vi "AssertValueByArrayTags.vi"(0 "VI Reference In":refnum<vi>, 1 "Test Label":string, 2 "delimiter (>>)":string=">>", 3 "Assert Only? (F)":bool, 5 "Control Path":string, 7 "Focus Item Tag":string[](array[string]), 11 "Error In":errorcluster, 12 "Assert Interval(10 ms)":u32=10, 13 "Timeout(5 sec)":dbl=5.0) -> (4 "VI Reference Out":refnum<vi>, 6 "Asserted Value":string[](array[string]), 15 "Error Out":errorcluster)   [LabVIEW 2016, in "Drona.lvlib" / "AssertControlValue.lvlib" / "AssertTree.lvlib"]
doc: "Asserts if the array of focus item tags for the multi-select tree control are equal.\n\nThe input control name is given as a string , incase of path, use delimiters inbetween the path.\nThis VI gets the value of the control, untill the value is equal to the input value."
uses:
  AssertTree.lvlib
  Get/GetControlRef/GetControlRefByPath.vi
  <vilib>/addons/_JKI Toolkits/Caraya/classes/Assert/Assert Equal Value_Variant.vi
  Get/GetControlRef/GetControlRef.lvlib
  <vilib>/addons/_JKI Toolkits/Caraya/classes/Assert/Assert.lvclass
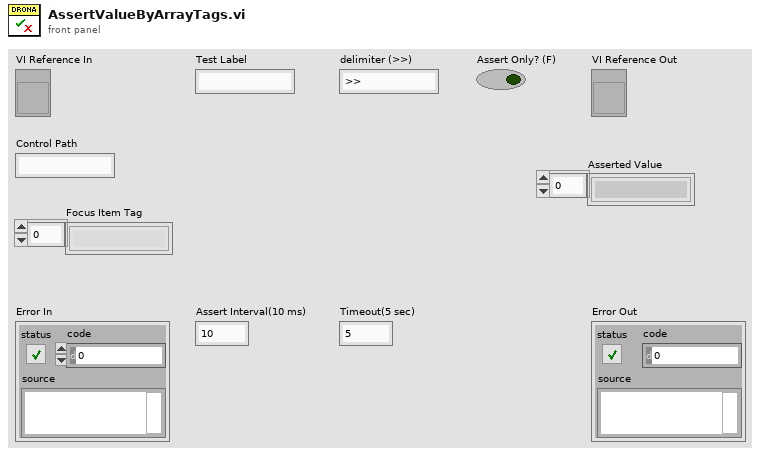
[diagram p1: front panel]
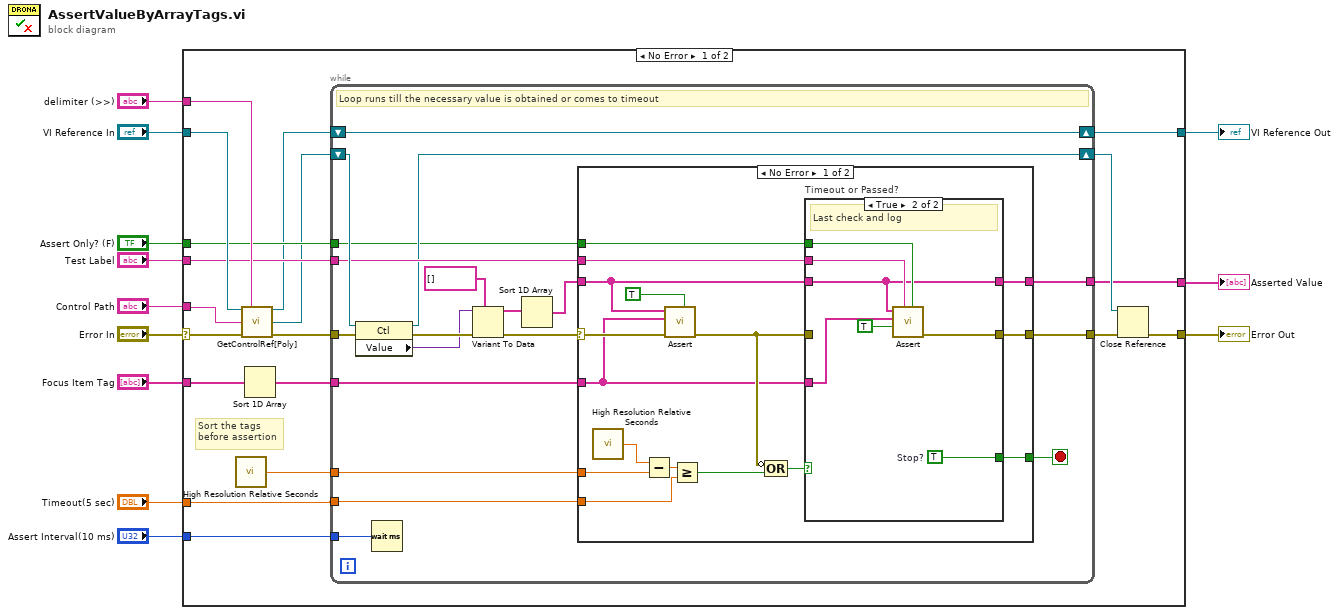
[diagram p0: block diagram]
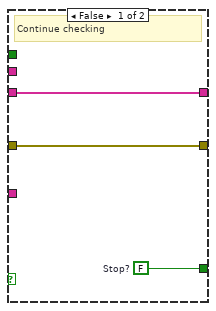
[diagram p2: hidden frame]
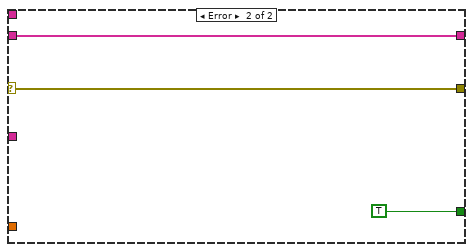
[diagram p3: hidden frame]
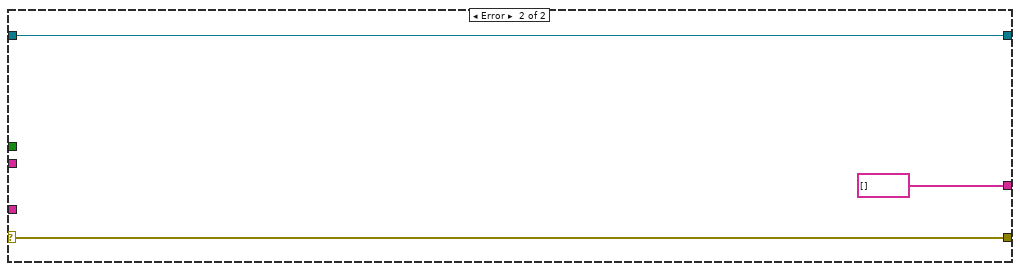
[diagram p4: hidden frame]
diagram:
  n1 = case shown="No Error" "Error In" {
    selector: "Error In" -> [w31 w82]
    tunnel: "Timeout(5 sec)" -> [w19 _]
    tunnel: [w16 w81] -> w11
    tunnel: "Focus Item Tag" -> [w21 _]
    tunnel: [w28 w82] -> w9
    tunnel: "Assert Interval(10 ms)" -> [w18 _]
    tunnel: "Test Label" -> [w25 _]
    tunnel: "VI Reference In" -> [w30 w81]
    tunnel: "Control Path" -> [w29 _]
    tunnel: "delimiter (>>)" -> [w27 _]
    tunnel: "Assert Only? (F)" -> [w24 _]
    tunnel: [w15 string[] []] -> w1
    frame No Error {
      # "Sort the tags\nbefore assertion"
      n2 = call <vilib>:"High Resolution Relative Seconds.vi"() -> ("relative seconds"=w20:dbl)
      n3 = call-poly "GetControlRef[Poly].vi"("VI Reference In"=w30, "delimiter (>>)"=w27, "Control Path"=w29, "error In"=w31) -> ("VI Reference Out"=w22:refnum<vi>, "Ctl Refnum"=w23:refnum<vi>, "error out"=w26:errorcluster)  [unwired: 9 in]
      n4 = Sort 1D Array(array=w21) -> (sorted array=w13:string[])
      n5 = while {
        tunnel: w13 -> [w34]
        tunnel: w19 -> [w49]
        tunnel: w20 -> [w50]
        tunnel: w26 -> [w44]
        tunnel: [w47] -> w14
        tunnel: w18 -> [w45]
        tunnel: w25 -> [w41]
        shift-right: [w42] -> w16
        shift-left: w22 -> [w42]
        shift-right: [w40] -> w17
        shift-left: w23 -> [w43]
        tunnel: w24 -> [w39]
        tunnel: [w38] -> w15
        stop <- w48 stop-if-true
        # "Loop runs till the necessary value is obtained or comes to timeout"
        n6 = property on="Property Node" class="Ctl"(reference=w43, error in=w44) -> (reference out=w40:refnum<vi>, error out=w46:errorcluster, "Value"=w36:variant)
        n7 = Wait (ms)(milliseconds to wait=w45) -> ()  [unwired: 1 out]
        n8 = Variant To Data(error in=w46, type=string[] [], Variant=w36) -> (data=w33:string[], error out=w37:errorcluster)
        n9 = Sort 1D Array(array=w33) -> (sorted array=w32:string[])
        n10 = case shown="No Error" w37 {
          selector: w37 -> [w62 w79]
          tunnel: w50 -> [w66 _]
          tunnel: w49 -> [w63 _]
          tunnel: [w53 TRUE] -> w48
          tunnel: [w54 w79] -> w47
          tunnel: w34 -> [w55 _]
          tunnel: w32 -> [w56 w77]
          tunnel: w41 -> [w61 _]
          tunnel: w39 -> [w52 _]
          tunnel: [w51 w77] -> w38
          frame No Error {
            n11 = call <vilib>:"High Resolution Relative Seconds.vi"() -> ("relative seconds"=w65:dbl)
            n12 = Subtract(x=w65, y=w66) -> (x-y=w64:dbl)
            n13 = call-poly <vilib>:"Assert.vi"("Assert Only? (F)"=TRUE, "error in (no error)"=w62, "Y"=w55, "X"=w56) -> ("error out"=w59:errorcluster)  [unwired: 7 in]
            n14 = Greater Or Equal?(x=w64, y=w63) -> (x >= y?=w60:bool)
            n15 = Compound Arithmetic op=OR(invert w59, w60) -> (w58:bool)
            n16 = case "Timeout or Passed?" shown="True" w58 {
              tunnel: w59 -> [w69 _]
              tunnel: w55 -> [_ w75]
              tunnel: w56 -> [w67 w70]
              tunnel: w61 -> [_ w76]
              tunnel: [w69 w74] -> w54
              tunnel: [w68 w73] -> w53
              tunnel: w52 -> [_ w71]
              tunnel: [w67 w70] -> w51
              frame False {
                w68 = FALSE  # Stop?
                # "Continue checking"
              }
              frame True {
                w73 = TRUE  # Stop?
                # "Last check and log"
                n17 = call-poly <vilib>:"Assert.vi"("Assert Only? (F)"=w71, "Label"=w76, "Register with caller test (F)"=TRUE, "Y"=w75, "X"=w70) -> ("error out"=w74:errorcluster)  [unwired: 6 in]
              }
            }
          }
          frame Error {
          }
        }
      }
      n18 = Close Reference(reference=w17, error in (no error)=w14) -> (error out=w28:errorcluster)
    }
    frame Error {
    }
  }
  "Error Out" <- w9
  "VI Reference Out" <- w11
  "Asserted Value" <- w1
